vi "calc_conveyor_module.vi"(0 "Ball Detector Count":i32, 1 "Reset":bool, 2 "Is Top Module":bool, 5 "Adjust Speed":dbl, 7 "Enable Conveyor":bool, 9 "Load Speed":dbl, 11 "Push Ball Out":bool, 12 "Ball is out":bool, 13 "Accept Balls?":bool=TRUE) -> (4 "Accepting Balls":bool, 6 "Conveyor Speed":dbl, 10 "Lifter Module State":T1)   [LabVIEW 2012]
uses:
  Conveyor module state.ctl
panel:
  in  "Max Ball\nMissing Count":dbl=5.0
  in  "Max Output Time":u32=1000
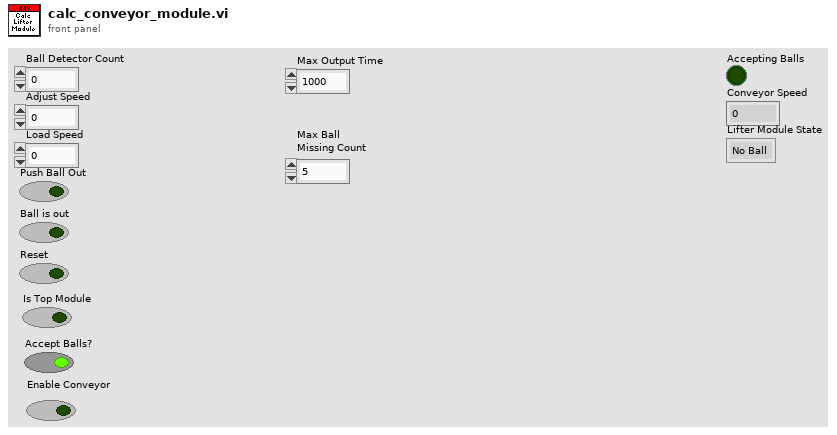
[diagram p1: front panel]
types:
  T1 = typedef "Conveyor module state.ctl" = enum16{"No Ball", "Has Ball", "Ball Below Hold", "Ball Above Hold", "Outputting Ball", "Reset"}
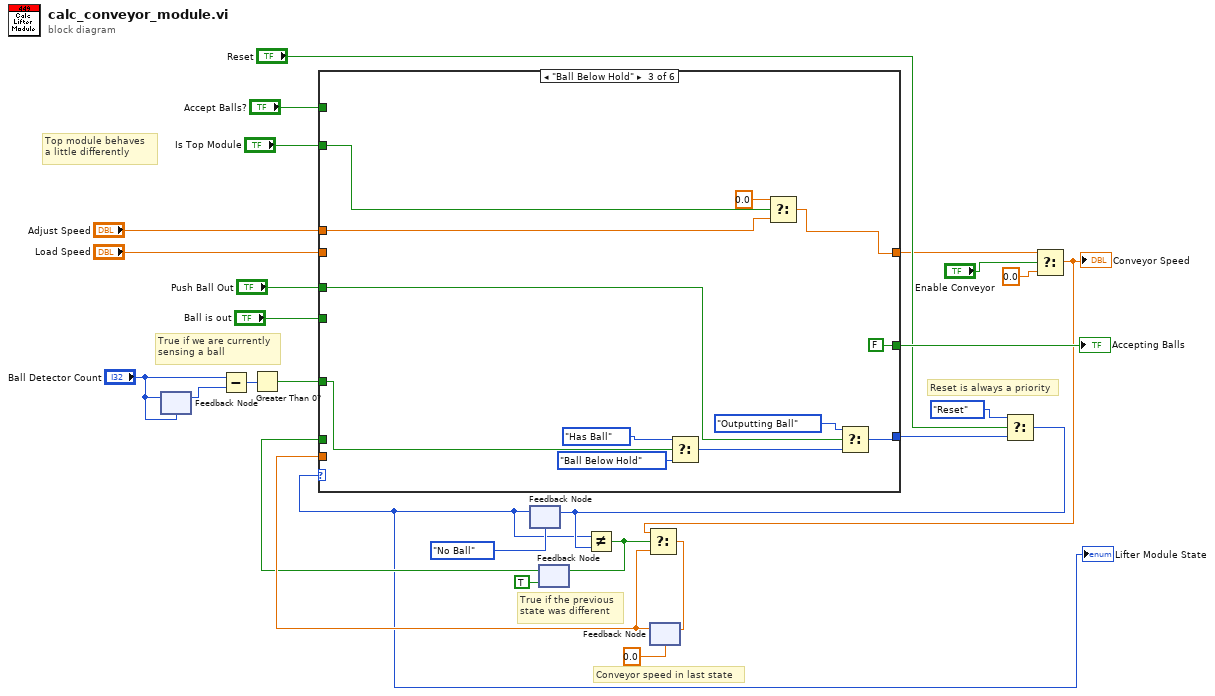
[diagram p0: block diagram]
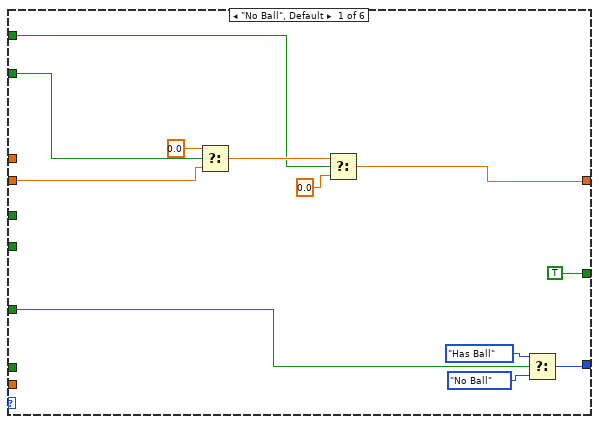
[diagram p2: hidden frame]
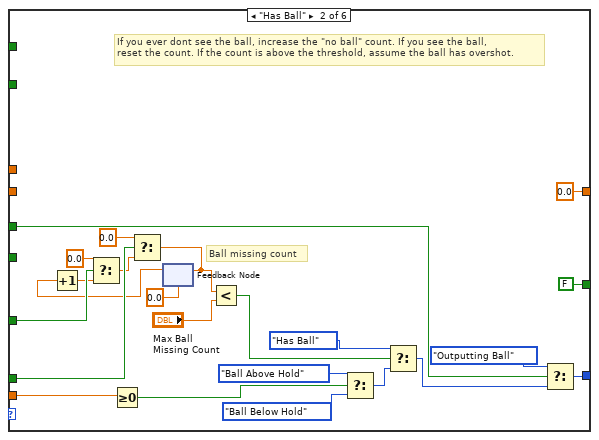
[diagram p3: hidden frame]
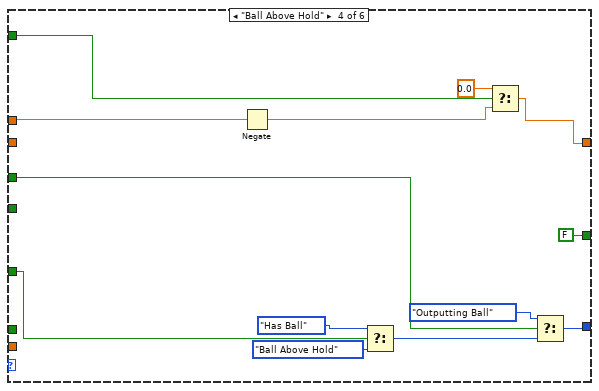
[diagram p4: hidden frame]
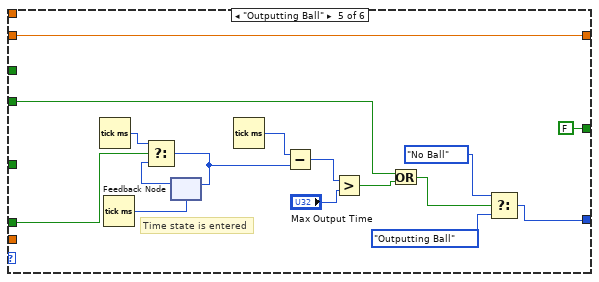
[diagram p5: hidden frame]
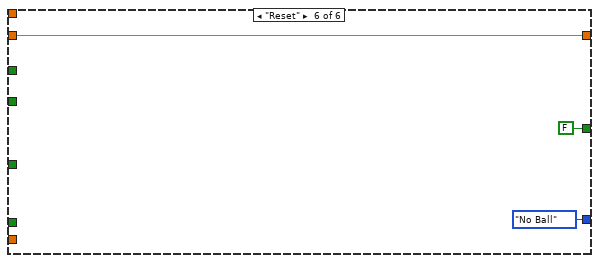
[diagram p6: hidden frame]
diagram:
  # "Top module behaves\na little differently"
  # "Reset is always a priority"
  # "True if the previous\nstate was different"
  # "Conveyor speed in last state"
  # "True if we are currently\nsensing a ball"
  n1 = feedback-in #1("Ball Detector Count") -> ()
  n2 = feedback #1("Ball Detector Count") -> (w27:i32)
  n3 = Subtract(x="Ball Detector Count", y=w27) -> (x-y=w26:i32)
  n4 = Greater Than 0?(x=w26) -> (x > 0?=w22:bool)
  n5 = feedback #2(Conveyor_module_state."No Ball" ("Conveyor Module State")) -> (w8:T1)
  "Lifter Module State" <- w8
  n6 = feedback #3(TRUE) -> (w14:bool)
  n7 = feedback #4(0.0 ("Load Speed")) -> (w17:dbl)
  n8 = case shown="\"Ball Below Hold\"" w8 {
    tunnel: [w38 w59 w74 w80 w88 Conveyor_module_state."No Ball" ("f")] -> w11
    tunnel: "Load Speed" -> [w34 _ _ _ w103 w105]
    tunnel: [w30 0.0 ("Load Speed") w65 w77 w103 w105] -> w3
    tunnel: "Adjust Speed" -> [_ _ w66 w83 _ _]
    tunnel: w22 -> [w39 w45 w70 w81 _ _]
    tunnel: [TRUE FALSE FALSE FALSE FALSE FALSE] -> w21
    tunnel: "Push Ball Out" -> [_ w60 w73 w82 _ _]
    tunnel: w17 -> [_ w54 _ _ _ _]
    tunnel: "Ball is out" -> [_ _ _ _ w92 _]
    tunnel: w14 -> [_ w49 _ _ w100 _]
    tunnel: "Is Top Module" -> [w33 _ w64 w76 _ _]
    tunnel: "Accept Balls?" -> [w29 _ _ _ _ _]
    frame "No Ball", Default {
      n9 = Select(t=0.0, s=w33, f=w34) -> (s? t:f=w31:dbl)
      n10 = Select(t=w31, s=w29, f=0.0 ("t")) -> (s? t:f=w30:dbl)
      n11 = Select(t=Conveyor_module_state."Has Ball" ("Conveyor Module State"), s=w39, f=Conveyor_module_state."No Ball" ("Conveyor Module State")) -> (s? t:f=w38:T1)
    }
    frame "Has Ball" {
      # "Ball missing count"
      # "If you ever dont see the ball, increase the \"no ball\" count. If you see the ball,\nreset the count. If the count is above the threshold, assume the ball has overshot."
      n12 = Greater Or Equal To 0?(x=w54) -> (x >= 0?=w53:bool)
      n13 = feedback #5(0.0 ("Load Speed")) -> (w43:dbl)
      n14 = Increment(x=w43) -> (x+1=w44:dbl)
      n15 = Select(t=0.0, s=w45, f=w44) -> (s? t:f=w47:dbl)
      n16 = Select(t=0.0, s=w49, f=w47) -> (s? t:f=w42:dbl)
      n17 = feedback-in #5(w42) -> ()
      n18 = Less?(x=w42, y="Max Ball\nMissing Count") -> (x < y?=w41:bool)
      n19 = Select(t=Conveyor_module_state."Ball Above Hold" ("Conveyor Module State"), s=w53, f=Conveyor_module_state."Ball Below Hold" ("Conveyor Module State")) -> (s? t:f=w55:T1)
      n20 = Select(t=Conveyor_module_state."Has Ball" ("Conveyor Module State"), s=w41, f=w55) -> (s? t:f=w57:T1)
      n21 = Select(t=Conveyor_module_state."Outputting Ball" ("Conveyor Module State"), s=w60, f=w57) -> (s? t:f=w59:T1)
    }
    frame "Ball Below Hold" {
      n22 = Select(t=Conveyor_module_state."Has Ball" ("Conveyor Module State"), s=w70, f=Conveyor_module_state."Ball Below Hold" ("Conveyor Module State")) -> (s? t:f=w71:T1)
      n23 = Select(t=0.0, s=w64, f=w66) -> (s? t:f=w65:dbl)
      n24 = Select(t=Conveyor_module_state."Outputting Ball" ("Conveyor Module State"), s=w73, f=w71) -> (s? t:f=w74:T1)
    }
    frame "Ball Above Hold" {
      n25 = Negate(x=w83) -> (-x=w78:dbl)
      n26 = Select(t=Conveyor_module_state."Has Ball" ("Conveyor Module State"), s=w81, f=Conveyor_module_state."Ball Above Hold" ("Conveyor Module State")) -> (s? t:f=w85:T1)
      n27 = Select(t=0.0, s=w76, f=w78) -> (s? t:f=w77:dbl)
      n28 = Select(t=Conveyor_module_state."Outputting Ball" ("Conveyor Module State"), s=w82, f=w85) -> (s? t:f=w80:T1)
    }
    frame "Outputting Ball" {
      # "Time state is entered"
      n29 = Tick Count (ms)() -> (millisecond timer value=w99:u32)
      n30 = Tick Count (ms)() -> (millisecond timer value=w101:u32)
      n31 = feedback #6(w101) -> (w98:u32)
      n32 = Select(t=w99, s=w100, f=w98) -> (s? t:f=w96:u32)
      n33 = feedback-in #6(w96) -> ()
      n34 = Tick Count (ms)() -> (millisecond timer value=w97:u32)
      n35 = Subtract(x=w97, y=w96) -> (x-y=w95:u32)
      n36 = Greater?(x=w95, y="Max Output Time") -> (0:w93:bool)
      n37 = Or(x=w92, y=w93) -> (x .or. y?=w91:bool)
      n38 = Select(t=Conveyor_module_state."No Ball" ("Conveyor Module State"), s=w91, f=Conveyor_module_state."Outputting Ball") -> (s? t:f=w88:T1)
    }
    frame "Reset" {
    }
  }
  "Accepting Balls" <- w21
  n39 = Select(t=Conveyor_module_state."Reset", s="Reset", f=w11) -> (s? t:f=w12:T1)
  n40 = feedback-in #2(w12) -> ()
  n41 = Not Equal?(x=w8, y=w12) -> (x != y?=w15:bool)
  n42 = feedback-in #3(w15) -> ()
  n43 = Select(t=w3, s="Enable Conveyor", f=0.0) -> (s? t:f=w4:dbl)
  "Conveyor Speed" <- w4
  n44 = Select(t=w4, s=w15, f=w17) -> (s? t:f=w18:dbl)
  n45 = feedback-in #4(w18) -> ()
